vi "DiffDriveExecute.vi"(8 "error in (no error)":errorcluster, 11 "Outputs\nEnabled":bool) -> (0 "error out":errorcluster)   [LabVIEW 2025]
uses:
  <vilib>/Rock Robotics/WPI/ThirdParty/Phoenix-LabVIEW/Motor Controller/Controls/CTRE_Phoenix_MotorControl_ControlMode.ctl
  <vilib>/Rock Robotics/WPI/ThirdParty/JAS_Junk/TrajLib/SimpleMotorFF_Calculate.vi
  DiffDriveGlobals.vi
  <vilib>/Rock Robotics/WPI/ThirdParty/JAS_Junk/TrajLib/Trajectory_Library.lvlib
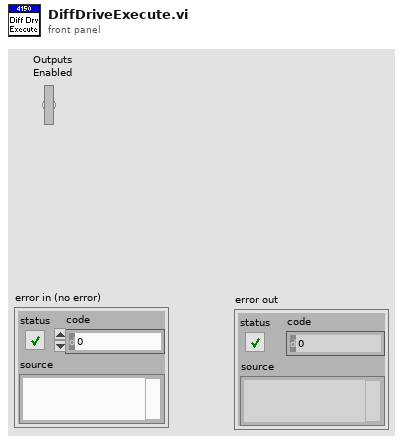
[diagram p1: front panel]
types:
  T1 = typedef "Trajectory_Library.lvlib/SIMPLE_MOTOR_FF.ctl" = cluster{"Ks":dbl, "Kv":dbl, "Ka":dbl, "KnInv":dbl}
  T2 = typedef "CTRE_Phoenix_MotorControl_ControlMode.ctl" = u16
  T3 = typedef "WPI_MotorControlDeviceRef.ctl" = cluster{"DeviceStatus":errorcluster, "Type":T4, "PWM":cluster{"PWM Channel":T5, "DeadBand":T6}, "CAN":cluster{"Device Number":u8, "SetOutput VI Ref":variant, "GetOutput VI Ref":variant, "Enable VI Ref":variant, "Disable VI Ref":variant, "Data":variant}, "Invert":bool, "DIO PWM":cluster{"PWM \"Enable\" Channel":T5, "DIOChannel":T7, "PWM Rate":dbl}}
  T4 = typedef "WPI_MotorControlType.ctl" = enum16{"PWM", "CAN", "DIO PWM"}
  T5 = typedef "FPGA_DIOPWMChannel.ctl" = enum8{"PWM 0", "PWM 1", "PWM 2", "PWM 3", "PWM 4", "PWM 5", "PWM 6", "PWM 7", "PWM 8", "PWM 9", "PWM MXP 0", "PWM MXP 1", "PWM MXP 2", "PWM MXP 3", "PWM MXP 4", "PWM MXP 5", "PWM MXP 6", "PWM MXP 7", "PWM MXP 8", "PWM MXP 9", "Invalid"}
  T6 = typedef "WPI_PWMDeadband.ctl" = cluster{"Name":string, "maxPositivePwm":i32, "minPositivePwm":i32, "centerPwm":i32, "maxNegativePwm":i32, "minNegativePwm":i32, "angularRange":u16}
  T7 = typedef "FPGA_DIOChannel.ctl" = enum8{"DIO 0", "DIO 1", "DIO 2", "DIO 3", "DIO 4", "DIO 5", "DIO 6", "DIO 7", "DIO 8", "DIO 9", "DIO MXP 0", "DIO MXP 1", "DIO MXP 2", "DIO MXP 3", "DIO MXP 4", "DIO MXP 5", "DIO MXP 6", "DIO MXP 7", "DIO MXP 8", "DIO MXP 9", "DIO MXP 10", "DIO MXP 11", "DIO MXP 12", "DIO MXP 13", "DIO MXP 14", "DIO MXP 15", "SPI Port CS1", "SPI Port CS2", "SPI Port CS3", "SPI Port MISO", "SPI Port MOSI", "Invalid"}
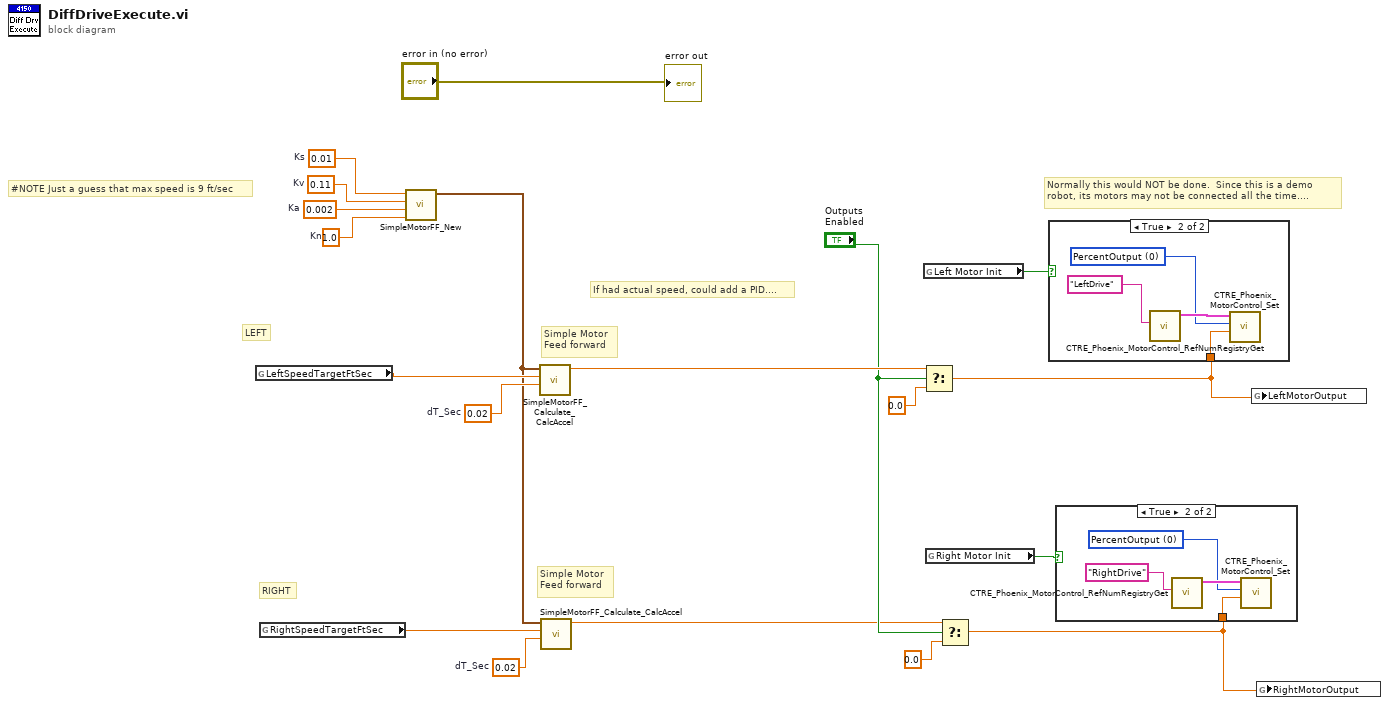
[diagram p0: block diagram]
diagram:
  w14 = 0.02  # dT_Sec
  w19 = 1.0  # Kn
  w18 = 0.02  # dT_Sec
  w17 = 0.01  # Ks
  w16 = 0.11  # Kv
  w15 = 0.002  # Ka
  # "Normally this would NOT be done.  Since this is a demo\nrobot, its motors may not be connected all the time...."
  # "If had actual speed, could add a PID...."
  # "#NOTE Just a guess that max speed is 9 ft/sec"
  # "Simple Motor\nFeed forward"
  # "Simple Motor\nFeed forward"
  # "RIGHT"
  # "LEFT"
  n1 = global read "DiffDriveGlobals.vi" "LeftSpeedTargetFtSec"() -> (w12:dbl)
  n2 = global read "DiffDriveGlobals.vi" "RightSpeedTargetFtSec"() -> (w13:dbl)
  n3 = call <vilib>:"SimpleMotorFF_New.vi"("Kn"=w19, "Ka"=w15, "Kv"=w16, "Ks"=w17) -> ("SIMPLE_MOTOR_FF"=w11:T1)  [unwired: 7 in]
  n4 = call <vilib>:"SimpleMotorFF_Calculate_CalcAccel.vi"("dT_Sec"=w18, "VelSp"=w12, "SIMPLE_MOTOR_FF"=w11) -> ("FeedForward"=w9:dbl)  [unwired: 8 in]
  n5 = call <vilib>:"SimpleMotorFF_Calculate_CalcAccel.vi"("dT_Sec"=w14, "VelSp"=w13, "SIMPLE_MOTOR_FF"=w11) -> ("FeedForward"=w4:dbl)  [unwired: 8 in]
  n6 = global read "DiffDriveGlobals.vi" "Left Motor Init"() -> (w2:bool)
  n7 = Select(t=w9, s="Outputs\nEnabled", f=0.0) -> (s? t:f=w8:dbl)
  n8 = global read "DiffDriveGlobals.vi" "Right Motor Init"() -> (w1:bool)
  n9 = Select(t=w4, s="Outputs\nEnabled", f=0.0) -> (s? t:f=w3:dbl)
  n10 = case shown="True" w2 {
    tunnel: w8 -> [_ w20]
    frame False {
    }
    frame True {
      w21 = T2 0 items=["PercentOutput"=0, "Position"=1, "Velocity"=2, "Current"=3, "Follower"=5, "MotionProfile"=6, "MotionMagic"=7, "MotionProfileArc"=10, "Disabled"=15] ("Control Mode")
      n11 = call <vilib>:"CTRE_Phoenix_MotorControl_RefNumRegistryGet.vi"("refnum name"="LeftDrive") -> ("PhoenixMotorControlDevRef"=w22:T3)  [unwired: 9 in, 1 out]
      n12 = call <vilib>:"CTRE_Phoenix_MotorControl_Set.vi"("Output"=w20, "Control Mode"=w21, "PhoenixMotorControlDevRef"=w22) -> ()  [unwired: 7 in, 2 out]
    }
  }
  n13 = case shown="True" w1 {
    tunnel: w3 -> [_ w25]
    frame False {
    }
    frame True {
      w24 = T2 0 items=["PercentOutput"=0, "Position"=1, "Velocity"=2, "Current"=3, "Follower"=5, "MotionProfile"=6, "MotionMagic"=7, "MotionProfileArc"=10, "Disabled"=15] ("Control Mode")
      n14 = call <vilib>:"CTRE_Phoenix_MotorControl_RefNumRegistryGet.vi"("refnum name"="RightDrive") -> ("PhoenixMotorControlDevRef"=w26:T3)  [unwired: 9 in, 1 out]
      n15 = call <vilib>:"CTRE_Phoenix_MotorControl_Set.vi"("Output"=w25, "Control Mode"=w24, "PhoenixMotorControlDevRef"=w26) -> ()  [unwired: 7 in, 2 out]
    }
  }
  n16 = global write "DiffDriveGlobals.vi" "LeftMotorOutput"(w8) -> ()
  n17 = global write "DiffDriveGlobals.vi" "RightMotorOutput"(w3) -> ()
  "error out" <- "error in (no error)"
